vi "Python_settings.vi"(2 "Task":enum16{"Read", "Write"}(ring), 4 "Settings in":T1) -> (1 "settings read":T1)   [LabVIEW 2025]
panel:
  out "error out":errorcluster
  in  "error in":errorcluster
  out "settings":path
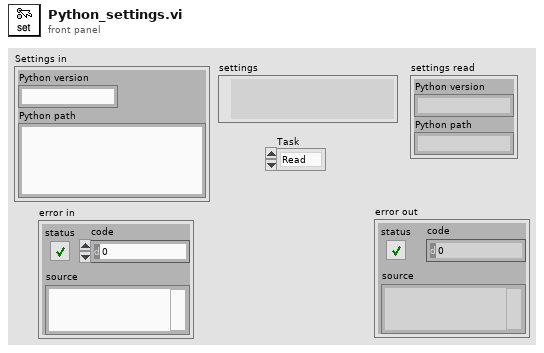
[diagram p1: front panel]
types:
  T1 = cluster{"Python version":string, "Python path":string}
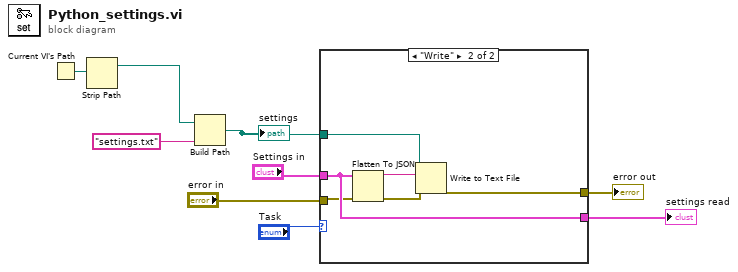
[diagram p0: block diagram]
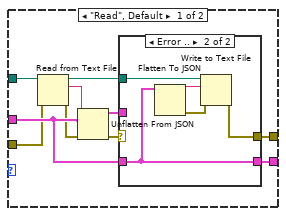
[diagram p2: hidden frame]
diagram:
  n1 = Current VI's Path() -> (path=w9:path)
  n2 = Strip Path(path=w9) -> (stripped path=w1:path)  [unwired: 1 out]
  n3 = Build Path(base path=w1, name or relative path="settings.txt") -> (appended path=w6:path)
  "settings" <- w6
  n4 = case shown="\"Write\"" "Task" {
    tunnel: w6 -> [w11 w31]
    tunnel: "Settings in" -> [w15 w29]
    tunnel: [w16 w29] -> w4
    tunnel: "error in" -> [w13 w28]
    tunnel: [w10 w26] -> w2
    frame "Read", Default {
      n5 = Read from Text File(file (use dialog)=w11, error in=w13) -> (text=w18:string, error out=w14:errorcluster)  [unwired: 2 in, 2 out]
      n6 = Unflatten From JSON(JSON string=w18, type and defaults=w15, error in (no error)=w14) -> (value=w17:T1, error out=w12:errorcluster)  [unwired: 4 in]
      n7 = case shown="Error .." w12 {
        selector: w12 -> [w19 _]
        tunnel: w17 -> [w20 _]
        tunnel: [w20 w23] -> w16
        tunnel: w15 -> [_ w23]
        tunnel: w11 -> [_ w25]
        tunnel: [w19 w24] -> w10
        frame No Error {
        }
        frame Error {
          n8 = Flatten To JSON(anything=w23) -> (JSON string=w22:string, 11:w21:errorcluster)  [unwired: 2 in]
          n9 = Write to Text File(file (use dialog)=w25, text=w22, error in=w21) -> (error out=w24:errorcluster)  [unwired: 1 in, 2 out]
        }
      }
    }
    frame "Write" {
      n10 = Flatten To JSON(anything=w29, error in (no error)=w28) -> (JSON string=w30:string, 11:w27:errorcluster)  [unwired: 1 in]
      n11 = Write to Text File(file (use dialog)=w31, text=w30, error in=w27) -> (error out=w26:errorcluster)  [unwired: 1 in, 2 out]
    }
  }
  "settings read" <- w4
  "error out" <- w2
